vi "DevFuncPan.vi"(8 "error in (no error)":errorcluster caption="entrée d'erreur (pas d'erreur)", 11 "Default.lvclass":refnum<class "Spex.lvclass">) -> (0 "error out":errorcluster caption="sortie d'erreur", 3 "Default.lvclass Out":refnum<class "Spex.lvclass">)   [LabVIEW 2019, in "Spex.lvclass"]
uses:
  Spex.lvclass
panel:
  out "4":dbl
  out "3":dbl
  out "5":dbl
  in  "2":dbl
  in  "1":dbl
  in  "Stop":bool
  in  "MiseAJour":bool
  out "Init Program":bool
  # "Base Device Panel"
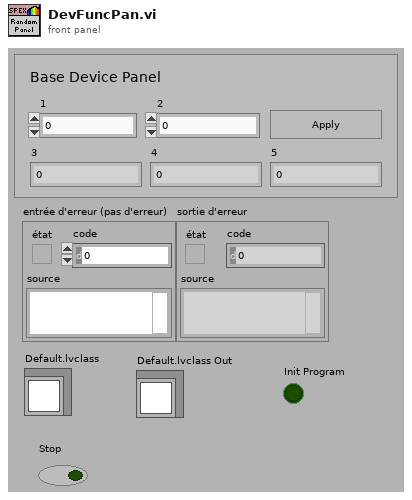
[diagram p1: front panel]
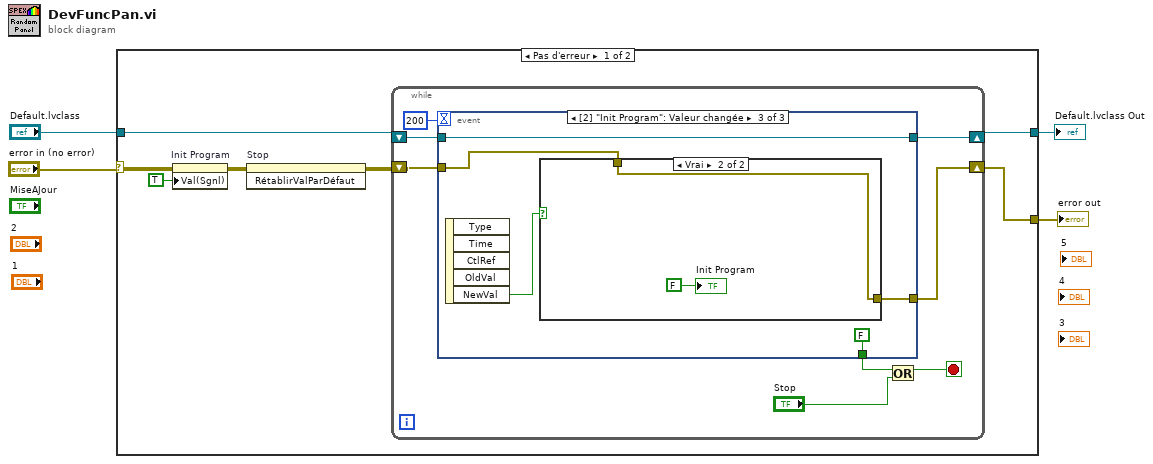
[diagram p0: block diagram]
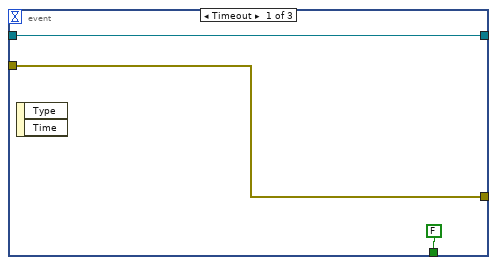
[diagram p2: hidden frame]
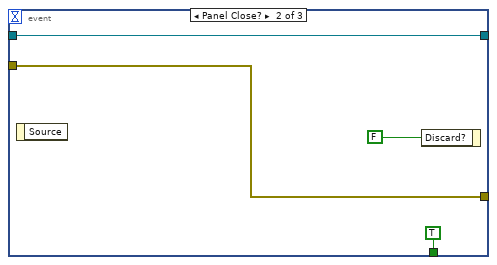
[diagram p3: hidden frame]
diagram:
  n1 = case shown="Pas d'erreur" "error in (no error)" {
    selector: "error in (no error)" -> [w8 w36]
    tunnel: [w11 w36] -> w3
    tunnel: "Default.lvclass" -> [w5 w35]
    tunnel: [w9 w35] -> w1
    frame No Error {
      n2 = property on="Init Program" class="Bool (strict)"(error in=w8, "Val(Sgnl)"=TRUE ("Valeur (Signalisation)")) -> (error out=w7:errorcluster)  [unwired: 1 in, 1 out]
      n3 = invoke on="Stop" class="Bool (strict)" method="RétablirValParDéfaut"(error in=w7) -> (error out=w6:errorcluster)  [unwired: 2 in, 2 out]
      n4 = while {
        shift-right: [w17] -> w11
        shift-left: w6 -> [w18]
        shift-right: [w14] -> w9
        shift-left: w5 -> [w16]
        stop <- w13 stop-if-true
        n5 = event shown="[2] \"Init Program\": Valeur changée" {
          selector: _ -> [_ _ _]
          dyn-events: _ -> [_ _ _]
          timeout: 200 -> [_ _ _]
          tunnel: w18 -> [w20 w24 w30]
          tunnel: [w20 w24 w29] -> w17
          tunnel: w16 -> [w21 w23 w28]
          tunnel: [FALSE TRUE FALSE] -> w15
          tunnel: [w21 w23 w28] -> w14
          event Timeout {
            n6 = event-data() -> ()  [unwired: 1 in, 2 out]
          }
          event Panel Close? {
            n7 = event-data() -> ()  [unwired: 1 in, 1 out]
            n8 = event-data("Discard?"=FALSE ("Rejeter ?")) -> ()  [unwired: 1 in, 1 out]
          }
          event "Init Program": Value Change {
            n9 = event-data() -> ("NewVal"=w31:bool)  [unwired: 1 in, 4 out]
            n10 = case shown="Vrai" w31 {
              tunnel: w30 -> [w32 w33]
              tunnel: [w32 w33] -> w29
              frame False {
              }
              frame True {
                "Init Program" <- FALSE
              }
            }
          }
        }
        n11 = Or(x=w15, y="Stop") -> (x .or. y?=w13:bool)
      }
    }
    frame Error {
    }
  }
  "error out" <- w3
  "Default.lvclass Out" <- w1
